vi "Size to Distance.vi"(1 "Numeric":dbl) -> (0 "Numeric 2":dbl)   [LabVIEW 2013]
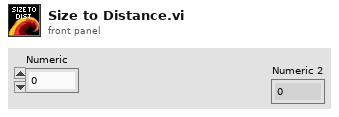
[diagram p1: front panel]
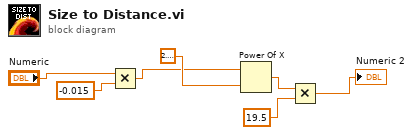
[diagram p0: block diagram]
diagram:
  n1 = Multiply(x="Numeric", y=-0.015) -> (x*y=w1:dbl)
  n2 = Power Of X(1:2.718281828459045, 2:w1) -> (0:w5:dbl)
  n3 = Multiply(x=w5, y=19.5) -> (x*y=→"Numeric 2":dbl)
